vi "Read Signal List.vi"(8 "error in (no error)":errorcluster, 11 "Performanced XNET CAN Signal Logger in":refnum<class "Performanced XNET CAN Logger.lvclass">) -> (0 "error out":errorcluster, 2 "data value":string[][](array[string]), 3 "Performanced XNET CAN Signal Logger out":refnum<class "Performanced XNET CAN Logger.lvclass">)   [LabVIEW 2021, in "Performanced XNET CAN Logger.lvlib" / "Performanced XNET CAN Logger.lvclass"]
uses:
  Performanced XNET CAN Logger.lvclass
  Performanced XNET CAN Logger.lvclass/Performanced XNET CAN Logger.ctl
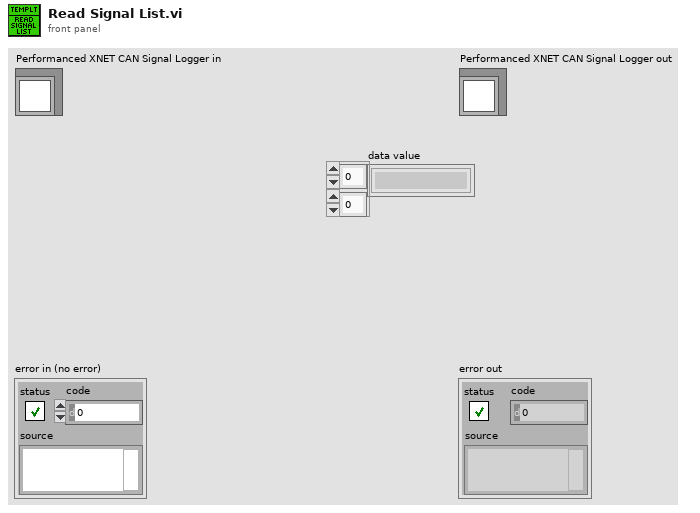
[diagram p1: front panel]
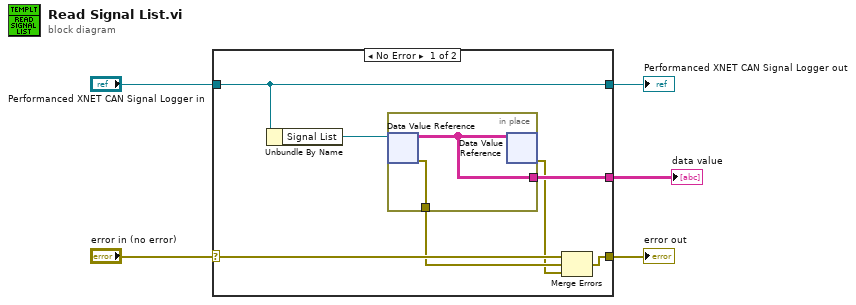
[diagram p0: block diagram]
diagram:
  n1 = case shown="No Error" "error in (no error)" {
    selector: "error in (no error)" -> [w12 w15]
    tunnel: [w8 w15] -> w4
    tunnel: [w11 w16] -> w2
    tunnel: "Performanced XNET CAN Signal Logger in" -> [w11 w16]
    tunnel: [w9 _] -> w1
    frame No Error {
      n2 = Unbundle By Name(w11) -> ("Signal List"=w10:refnum<data-value>)
      n3 = in-place {
        in-place-border: [w14] -> w7
        in-place-border: [w13] -> w9
        n4 = in-place-dvr #1(w10) -> (w13:string[][], w14:errorcluster)
        n5 = in-place-dvr #1(w13) -> (w6:errorcluster)  [unwired: 1 out]
      }
      n6 = Merge Errors(w12, w7, w6) -> (w8:errorcluster)
    }
    frame Error {
    }
  }
  "error out" <- w4
  "Performanced XNET CAN Signal Logger out" <- w2
  "data value" <- w1
